vi "Lines array to Corner Array.vi"(11 "Lines":T2[](array[typedef])) -> (3 "Corners":T1[](array[typedef]))   [LabVIEW 2017]
uses:
  Vector Library/Line.ctl
  Vector Library/Vector.ctl
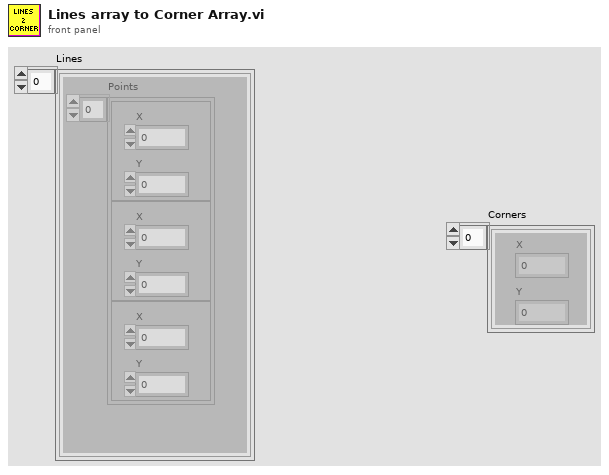
[diagram p1: front panel]
types:
  T1 = typedef "Vector.ctl" = cluster{"X":dbl, "Y":dbl}
  T2 = typedef "Line.ctl" = cluster{"Points":T1[]}
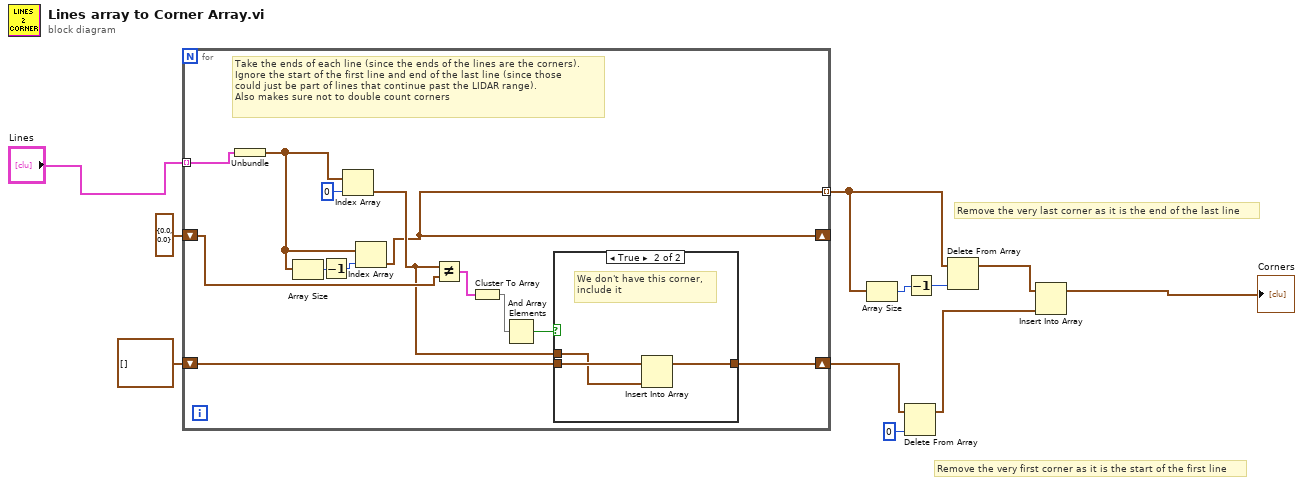
[diagram p0: block diagram]
diagram:
  # "Remove the very first corner as it is the start of the first line"
  # "Remove the very last corner as it is the end of the last line"
  n1 = for {
    tunnel: "Lines" -> [w24] mode=indexing
    tunnel: [w13] -> w8 mode=indexing
    shift-right: [w13] -> _
    shift-left: T1 {"X"=0.0, "Y"=0.0} ("Start") -> [w20]
    shift-right: [w15] -> w6
    shift-left: T1[] [] -> [w16]
    # "Take the ends of each line (since the ends of the lines are the corners).\nIgnore the start of the first line and end of the last line (since those\ncould just be part of lines that continue past the LIDAR range).\nAlso makes sure not to double count corners"
    n2 = Unbundle(w24) -> ("Points"=w21:T1[])
    n3 = Array Size(array=w21) -> (size(s)=w22:i32)
    n4 = Decrement(x=w22) -> (x-1=w12:i32)
    n5 = Index Array(array=w21, index=0) -> (element=w14:T1)
    n6 = Index Array(array=w21, index=w12) -> (element=w13:T1)
    n7 = Not Equal?(x=w14, y=w20) -> (x != y?=w19:cluster{"X":bool, "Y":bool})
    n8 = Cluster To Array(cluster=w19) -> (array=w17:bool[])
    n9 = And Array Elements(Boolean array=w17) -> (logical AND=w18:bool)
    n10 = case shown="True" w18 {
      tunnel: w16 -> [w25 w28]
      tunnel: [w25 w26] -> w15
      tunnel: w14 -> [_ w27]
      frame False {
        # "We already have this corner,\ndo not add it"
      }
      frame True {
        # "We don't have this corner,\ninclude it"
        n11 = Insert Into Array(array=w28, new element=w27) -> (w26:T1[])  [unwired: 1 in]
      }
    }
  }
  n12 = Array Size(array=w8) -> (size(s)=w9:i32)
  n13 = Delete From Array(array=w6, index=0) -> (array with subset deleted=w4:T1[])  [unwired: 1 in, 1 out]
  n14 = Decrement(x=w9) -> (x-1=w7:i32)
  n15 = Delete From Array(array=w8, index=w7) -> (array with subset deleted=w11:T1[])  [unwired: 1 in, 1 out]
  n16 = Insert Into Array(array=w11, new element=w4) -> (→"Corners":T1[])  [unwired: 1 in]
